vi "prueba2_240.vi"() -> ()   [LabVIEW 2011]
panel:
  out "Mayor a 40":bool
  out "Contado>40":dbl
  out "TemperaturaPromedio":dbl
  out "TemperaturaMenor":dbl
  out "TemperaturaMayor":dbl
  out "Temperatura":i32(slide) scale=0.0..60.0
  # "Se tiene que generar una temperatura  entre 1-60, luego deberá de encender un\nled cada vez, que la temperatura sea mayor a 40 y deberá de contarla.\nSe tiene que obtener el numero mayor y menor .\nLa temperatura promedi solo se obtiene de los temperaturas mayores a 30.\nHacerlo 5 veces, usar el ciclo for."
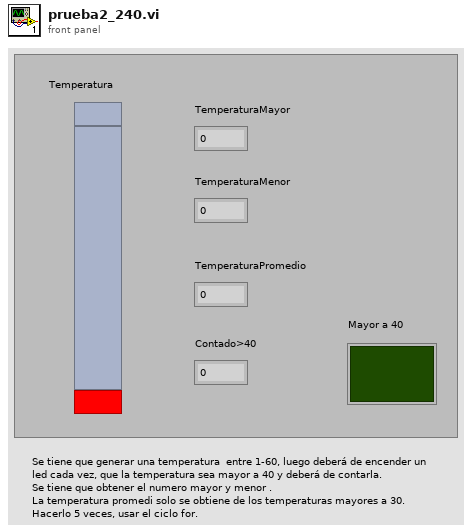
[diagram p1: front panel]
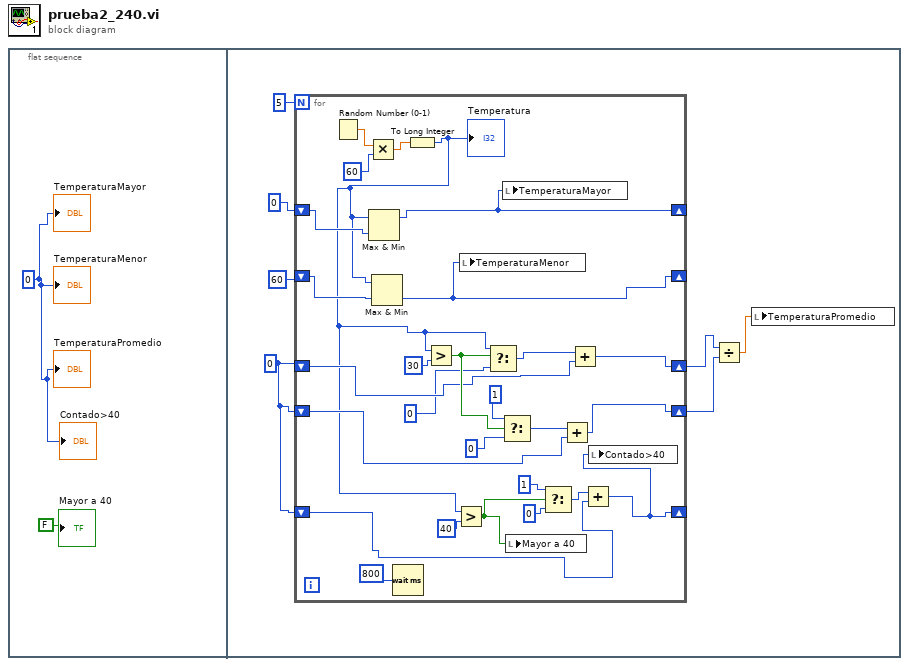
[diagram p0: block diagram]
diagram:
  n1 = flat-sequence {
    frame #0 {
      w2 = 0
      "TemperaturaMayor" <- w2
      "TemperaturaMenor" <- w2
      "TemperaturaPromedio" <- w2
      "Contado>40" <- w2
      "Mayor a 40" <- FALSE
    }
    frame #1 {
      w3 = 0
      n2 = for {
        N: 5 -> [_]
        shift-right: [w31] -> _
        shift-left: 0 -> [w32]
        shift-right: [w30] -> _
        shift-left: 60 -> [w33]
        shift-right: [w22] -> w6
        shift-left: w3 -> [w25]
        shift-right: [w19] -> w4
        shift-left: w3 -> [w21]
        shift-right: [w11] -> _
        shift-left: w3 -> [w12]
        n3 = Random Number (0-1)() -> (number: 0 to 1=w35:dbl)
        n4 = Multiply(x=w35, y=60) -> (x*y=w34:dbl)
        n5 = Wait (ms)(milliseconds to wait=800) -> ()  [unwired: 1 out]
        n6 = To Long Integer(number=w34) -> (32bit integer=w18:i32)
        "Temperatura" <- w18
        n7 = Max & Min(x=w18, y=w32) -> (max(x,y)=w31:i32)  [unwired: 1 out]
        n8 = Max & Min(x=w18, y=w33) -> (min(x,y)=w30:i32)  [unwired: 1 out]
        n9 = Greater?(x=w18, y=30) -> (0:w28:bool)
        n10 = Greater?(x=w18, y=40) -> (0:w16:bool)
        n11 = local write "TemperaturaMenor"(w30) -> ()
        n12 = Select(t=w18, s=w28, f=0) -> (s? t:f=w23:i32)
        n13 = Select(t=1, s=w28, f=0 ("t")) -> (s? t:f=w20:i32)
        n14 = local write "TemperaturaMayor"(w31) -> ()
        n15 = local write "Mayor a 40"(w16) -> ()
        n16 = Select(t=1, s=w16, f=0 ("t")) -> (s? t:f=w13:i32)
        n17 = Add(x=w20, y=w21) -> (x+y=w19:i32)
        n18 = Add(x=w23, y=w25) -> (x+y=w22:i32)
        n19 = Add(x=w13, y=w12) -> (x+y=w11:i32)
        n20 = local write "Contado>40"(w11) -> ()
      }
      n21 = Divide(x=w6, y=w4) -> (x/y=w5:dbl)
      n22 = local write "TemperaturaPromedio"(w5) -> ()
    }
  }
